vi "GetPolyScopeVersion.vi"(0 "Universal Robot.lvclass in":refnum<class "Universal Robot.lvclass">, 5 "error in (no error)":errorcluster) -> (14 "Universal Robot.lvclass out":refnum<class "Universal Robot.lvclass">, 15 "polyscopeVersion":string, 19 "error out":errorcluster)   [LabVIEW 2016, in "Universal Robot.lvclass"]
uses:
  Universal Robot/Universal Robot.lvclass
  Universal Robot/PolyScopeVersion.ctl
  Universal Robot/Universal Robot.lvclass/Universal Robot.ctl
  <vilib>/regexp/Match Regular Expression.xnode
  Dashboard Server.lvclass
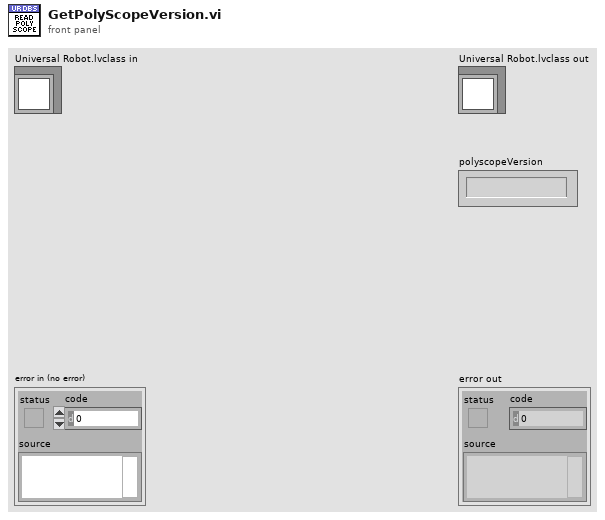
[diagram p1: front panel]
types:
  T1 = typedef "Universal Robot.lvclass/PolyScopeVersion.ctl" = cluster{"Major":i32, "Minor":i32, "Fix":i32, "Build":i32}
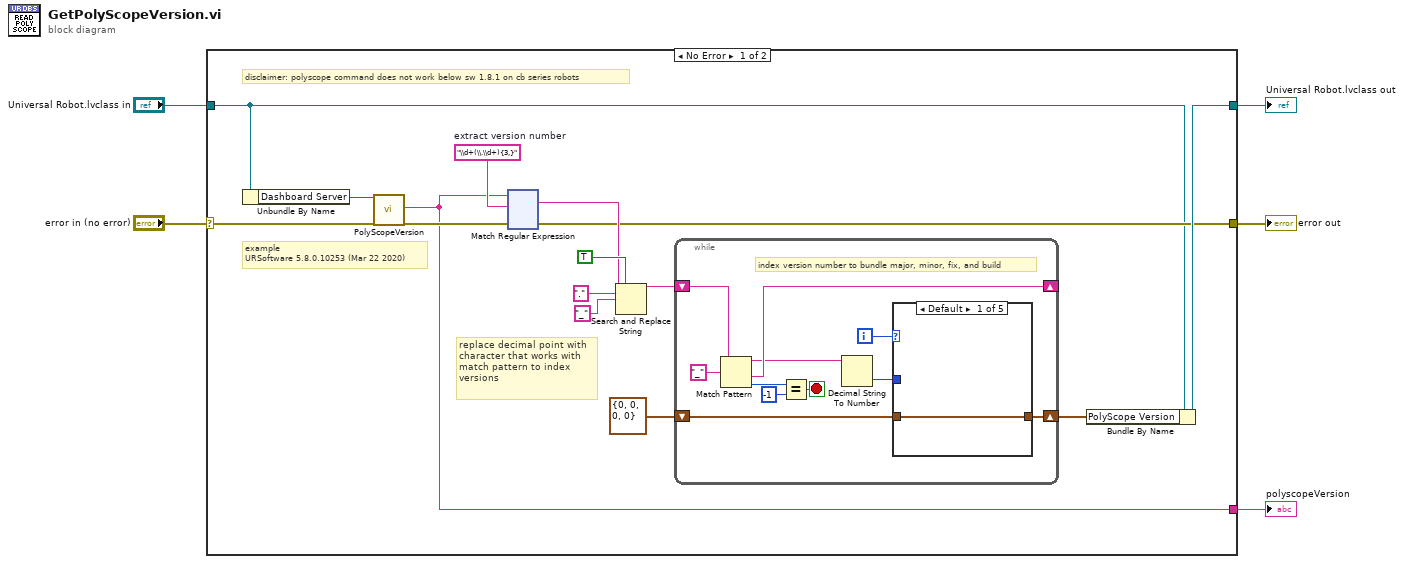
[diagram p0: block diagram]
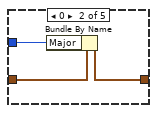
[diagram p2: hidden frame]
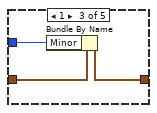
[diagram p3: hidden frame]
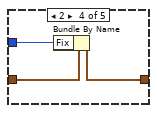
[diagram p4: hidden frame]
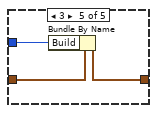
[diagram p5: hidden frame]
diagram:
  n1 = case shown="No Error" "error in (no error)" {
    selector: "error in (no error)" -> [w9 w160]
    tunnel: [w13 w160] -> w4
    tunnel: "Universal Robot.lvclass in" -> [w12 w159]
    tunnel: [w6 _] -> w3
    tunnel: [w19 w159] -> w1
    frame No Error {
      w20 = "\\d+(\\.\\d+){3,}"  # extract version number
      # "disclaimer: polyscope command does not work below sw 1.8.1 on cb series robots"
      # "replace decimal point with character that works with match pattern to index versions"
      # "example\nURSoftware 5.8.0.10253 (Mar 22 2020)"
      n2 = Unbundle By Name(w12) -> ("Dashboard Server"=w8:refnum<class "Dashboard Server.lvclass">)
      n3 = call-dynamic "PolyScopeVersion.vi"("DashboardServer in"=w8, "error in (no error)"=w9) -> ("PolyScopeVersion"=w6:string, "error out"=w7:errorcluster)  [unwired: 15 in, 1 out]
      n4 = xnode "Match Regular Expression"("input string"=w6, "regular expression"=w20, "error in"=w7) -> ("whole match"=w14:string, "error out"=w13:errorcluster)  [unwired: 3 in, 3 out]
      n5 = Search and Replace String(replace all?=TRUE ("replace all? (F)"), input string=w14, search string=".", replace string="_" ("replace string (\"\")")) -> (result string=w18:string)  [unwired: 4 in, 3 out]
      n6 = while {
        shift-right: [w30] -> _
        shift-left: w18 -> [w26]
        shift-right: [w21] -> w10
        shift-left: T1 {"Major"=0, "Minor"=0, "Fix"=0, "Build"=0} ("PolyScope Version") -> [w24]
        i -> [w25]
        stop <- w27 stop-if-true
        # "index version number to bundle major, minor, fix, and build"
        n7 = Match Pattern(string=w26, regular expression="_") -> (before substring=w23:string, after substring=w30:string, offset past match=w29:i32)  [unwired: 1 in, 1 out]
        n8 = Equal?(x=w29, y=-1) -> (x = y?=w27:bool)
        n9 = Decimal String To Number(string=w23) -> (number=w22:i32)  [unwired: 2 in, 1 out]
        n10 = case shown="Default" w25 {
          tunnel: w24 -> [w32 w35 w38 w41 w44]
          tunnel: w22 -> [_ w34 w37 w40 w43]
          tunnel: [w32 w33 w36 w39 w42] -> w21
          frame Default {
          }
          frame 0 {
            n11 = Bundle By Name(cluster=w35, "Major"=w34) -> (w33:T1)
          }
          frame 1 {
            n12 = Bundle By Name(cluster=w38, "Minor"=w37) -> (w36:T1)
          }
          frame 2 {
            n13 = Bundle By Name(cluster=w41, "Fix"=w40) -> (w39:T1)
          }
          frame 3 {
            n14 = Bundle By Name(cluster=w44, "Build"=w43) -> (w42:T1)
          }
        }
      }
      n15 = Bundle By Name(cluster=w12, "PolyScope Version"=w10) -> (w19:refnum<class "Universal Robot.lvclass">)
    }
    frame Error {
    }
  }
  "error out" <- w4
  "polyscopeVersion" <- w3
  "Universal Robot.lvclass out" <- w1
